vi "Generate Error.vi"(7 "Is Warning? (False)":bool, 8 "Error In":errorcluster, 9 "Arguments":string[](array[string]), 10 "Error Type":T5, 11 "LINX Device Config":T1) -> (0 "Error Out":errorcluster, 3 "LINX Device Config":T1)   [LabVIEW 2013, in "LVH-LINX.lvlib"]
doc: "Generate a LINX error based on the Error Type input."
uses:
  <vilib>/LabVIEW Hacker/LINX/LVH-LINX.lvlib
  <vilib>/LabVIEW Hacker/LINX/Private/Type Defs/Error Type.ctl
  <vilib>/LabVIEW Hacker/LINX/Private/Device/Type Defs/LINX Device Config.ctl
  <vilib>/LabVIEW Hacker/LINX/Private/Type Defs/Interface.ctl
  <vilib>/LabVIEW Hacker/LINX/Private/Device/Type Defs/TCP Config.ctl
  <vilib>/LabVIEW Hacker/LINX/Private/Type Defs/Device Family.ctl
  <vilib>/LabVIEW Hacker/LINX/Private/Device/Device.lvlib
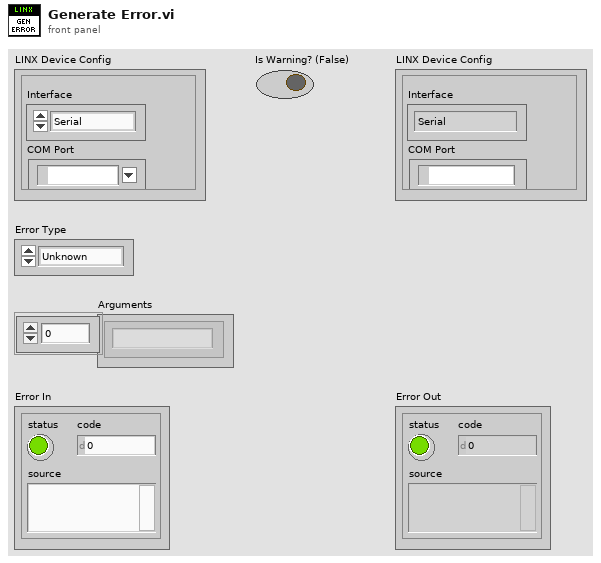
[diagram p1: front panel]
types:
  T1 = typedef "LVH-LINX.lvlib/Device.lvlib/LINX Device Config.ctl" = cluster{"Interface":T2, "COM Port":refnum<visa-resource-name>, "TCP Configuration":T3, "Device Family":T4, "Device ID":u8, "Device Name":string, "TCP Ref":refnum<k5>}
  T2 = typedef "LVH-LINX.lvlib/Interface.ctl" = enum16{"Serial", "TCP"}
  T3 = typedef "LVH-LINX.lvlib/Device.lvlib/TCP Config.ctl" = cluster{"IP Address":string, "Port":u16}
  T4 = typedef "LVH-LINX.lvlib/Device Family.ctl" = enum8{"National Instruments", "Digilent", "Arduino"}
  T5 = typedef "LVH-LINX.lvlib/Error Type.ctl" = enum16{"Unknown", "Timeout", "Corrupt Return Packet", "Unable To Connect", "Command Not Supported", "Channel DNE", "Invalid COM Config"}
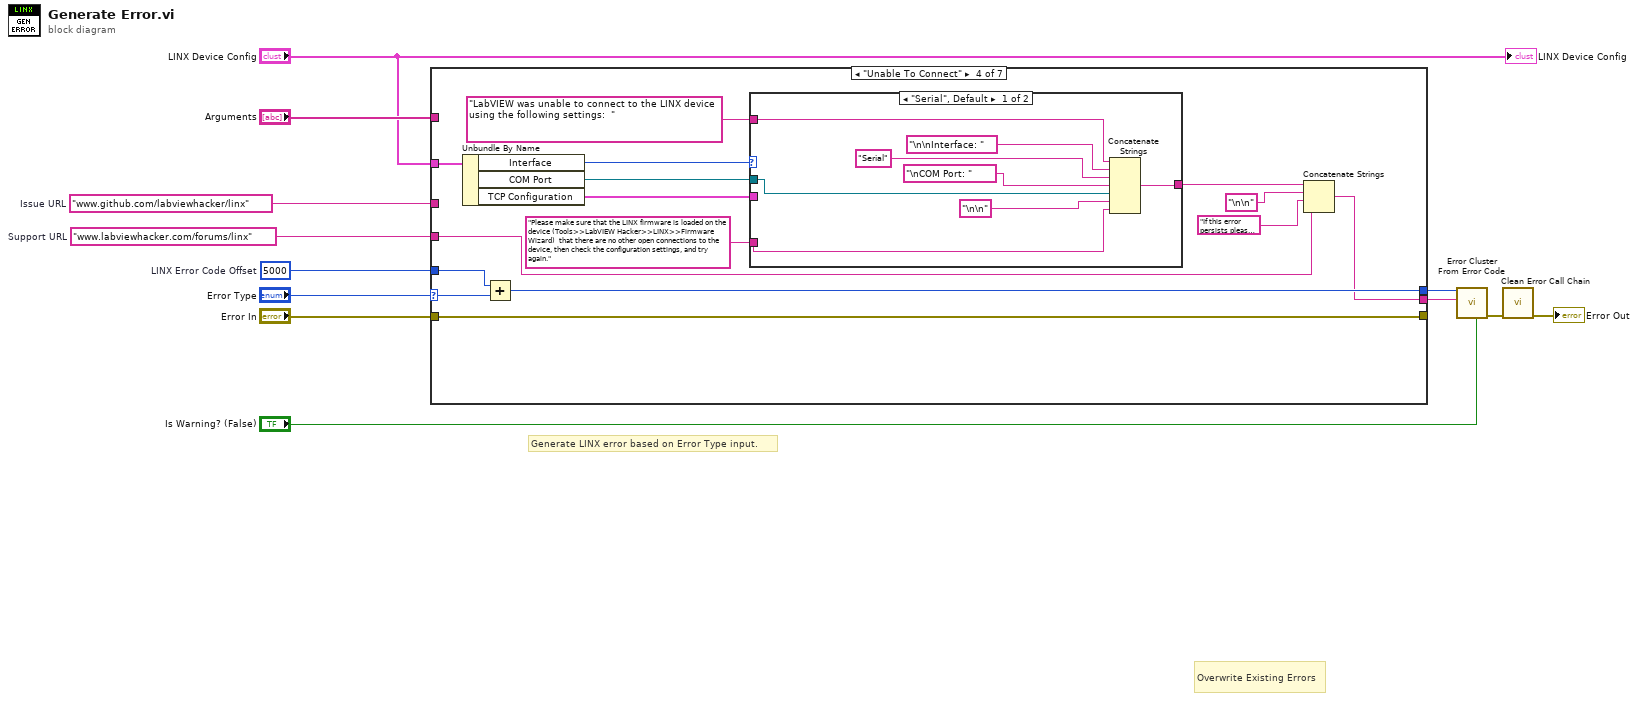
[diagram p0: block diagram]
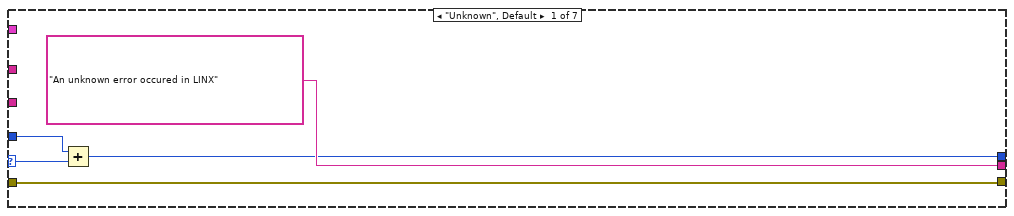
[diagram p2: hidden frame]
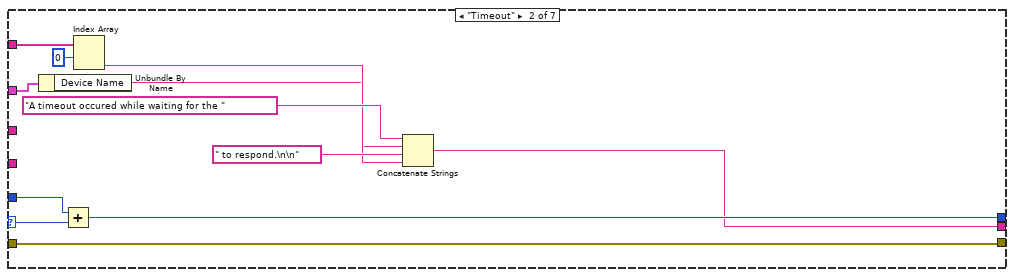
[diagram p3: hidden frame]
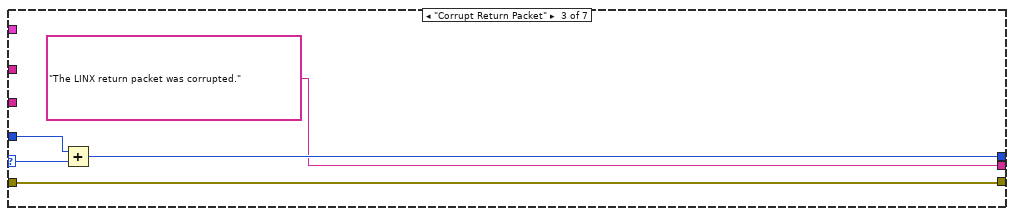
[diagram p4: hidden frame]
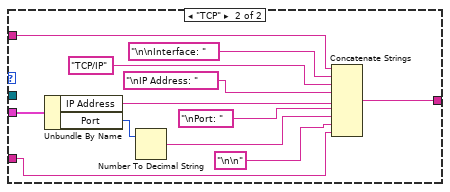
[diagram p5: hidden frame]
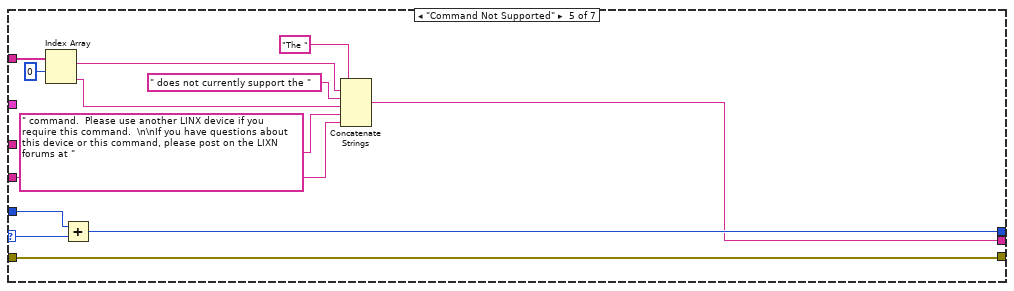
[diagram p6: hidden frame]
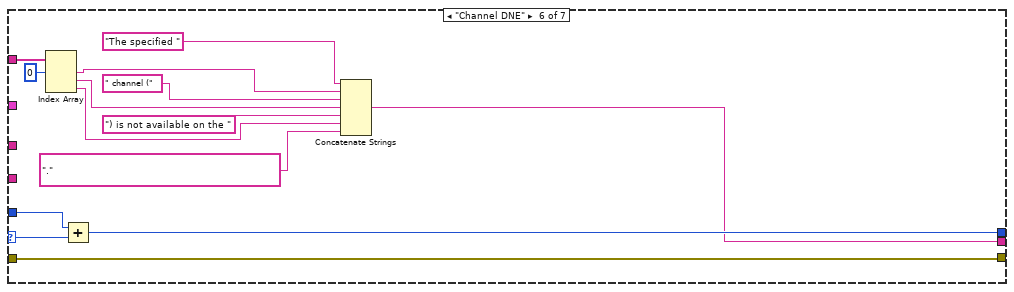
[diagram p7: hidden frame]
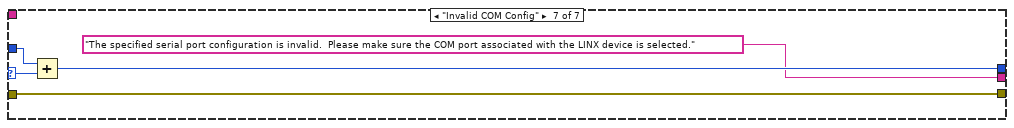
[diagram p8: hidden frame]
diagram:
  w3 = "www.labviewhacker.com/forums/linx"  # Support URL
  w6 = "www.github.com/labviewhacker/linx"  # Issue URL
  w11 = 5000  # LINX Error Code Offset
  # "Overwrite Existing Errors"
  # "Generate LINX error based on Error Type input."
  n1 = case shown="\"Unable To Connect\"" "Error Type" {
    selector: "Error Type" -> [w16 w28 w33 w48 w81 w95 w100]
    tunnel: "Error In" -> [w15 w26 w30 w47 w80 w94 w97]
    tunnel: [w15 w26 w30 w47 w80 w94 w97] -> _
    tunnel: w11 -> [w17 w29 w34 w49 w82 w96 w101]
    tunnel: ["An unknown error occured in LINX" ("error message (\"\")") w24 "The LINX return packet was corrupted." ("error message (\"\")") w36 w76 w92 "The specified serial port configuration is invalid.  Please make sure the COM port associated with the LINX device is selected."] -> w9
    tunnel: [w13 w27 w32 w46 w79 w93 w99] -> w8
    tunnel: w6 -> [_ _ _ _ _ _ _]
    tunnel: "Arguments" -> [_ w23 _ _ w74 w91 _]
    tunnel: "LINX Device Config" -> [_ w19 _ w45 _ _ _]
    tunnel: w3 -> [_ _ _ w35 w70 _ _]
    frame "Unknown", Default {
      n2 = Add(x=w17, y=w16) -> (x+y=w13:i32)
    }
    frame "Timeout" {
      n3 = Unbundle By Name(w19) -> ("Device Name"=w18:string)
      n4 = Add(x=w29, y=w28) -> (x+y=w27:i32)
      n5 = Index Array(array=w23, index #1=0 ("index")) -> (element #2=w20:string)  [unwired: 1 in, 1 out]
      n6 = Concatenate Strings("A timeout occured while waiting for the " ("error message (\"\")"), w18, " to respond.\n\n" ("string"), w20) -> (w24:string)
    }
    frame "Corrupt Return Packet" {
      n7 = Add(x=w34, y=w33) -> (x+y=w32:i32)
    }
    frame "Unable To Connect" {
      n8 = Unbundle By Name(w45) -> ("Interface"=w44:T2, "COM Port"=w40:refnum<visa-resource-name>, "TCP Configuration"=w43:T3)
      n9 = Add(x=w49, y=w48) -> (x+y=w46:i32)
      n10 = case shown="\"Serial\", Default" w44 {
        tunnel: w43 -> [_ w69]
        tunnel: "LabVIEW was unable to connect to the LINX device using the following settings:  " ("error message (\"\")") -> [w54 w65]
        tunnel: "Please make sure that the LINX firmware is loaded on the device (Tools>>LabVIEW Hacker>>LINX>>Firmware Wizard)  that there are no other open connections to the device, then check the configuration settings, and try again." -> [w50 w59]
        tunnel: [w52 w58] -> w39
        tunnel: w40 -> [w53 _]
        frame "Serial", Default {
          n11 = Concatenate Strings(w54, "\n\nInterface: " ("string"), "Serial" ("string"), "\nCOM Port: " ("string"), w53, "\n\n" ("string"), w50) -> (w52:string)
        }
        frame "TCP" {
          n12 = Unbundle By Name(w69) -> ("IP Address"=w63:string, "Port"=w68:u16)
          n13 = Number To Decimal String(number=w68) -> (decimal integer string=w61:string)  [unwired: 1 in]
          n14 = Concatenate Strings(w65, "\n\nInterface: " ("string"), "TCP/IP" ("string"), "\nIP Address: " ("string"), w63, "\nPort: " ("string"), w61, "\n\n" ("string"), w59) -> (w58:string)
        }
      }
      n15 = Concatenate Strings(w39, "\n\n" ("string"), "If this error persists please search, then post on the LINX forums at " ("error message (\"\")"), w35) -> (w36:string)
    }
    frame "Command Not Supported" {
      n16 = Index Array(array=w74, index #1=0 ("index")) -> (element #1=w72:string, element #2=w71:string)  [unwired: 1 in]
      n17 = Add(x=w82, y=w81) -> (x+y=w79:i32)
      n18 = Concatenate Strings("The " ("string"), w72, " does not currently support the " ("string"), w71, " command.  Please use another LINX device if you require this command.  \n\nIf you have questions about this device or this command, please post on the LIXN forums at " ("string"), w70) -> (w76:string)
    }
    frame "Channel DNE" {
      n19 = Index Array(array=w91, index #1=0 ("index")) -> (element #1=w89:string, element #2=w88:string, element #3=w84:string)  [unwired: 2 in]
      n20 = Add(x=w96, y=w95) -> (x+y=w93:i32)
      n21 = Concatenate Strings("The specified ", w89, " channel (" ("string"), w88, ") is not available on the " ("string"), w84, "." ("string")) -> (w92:string)
    }
    frame "Invalid COM Config" {
      n22 = Add(x=w101, y=w100) -> (x+y=w99:i32)
    }
  }
  n23 = call <vilib>:"Error Cluster From Error Code.vi"("is warning? (False)"="Is Warning? (False)", "error message (\"\")"=w9, "error code (0)"=w8) -> ("error out"=w2:errorcluster)  [unwired: 6 in]
  n24 = call <vilib>:"Clean Error Call Chain.vi"("Error In"=w2) -> ("Error Out"=→"Error Out":errorcluster)  [unwired: 10 in]
  "LINX Device Config" <- "LINX Device Config"
